vi "TREE_Get Sub Items.vi"(8 "error in":errorcluster, 10 "Par Tag":string, 11 "TreeRef":refnum<vi>) -> (0 "error out":errorcluster, 1 "Items":string[](array[string]), 2 "Tags":string[](array[string]), 3 "TreeRef":refnum<vi>)   [LabVIEW 2016]
doc: "Get sub items through input parent tag."
panel:
  # "Input"
  # "Output"
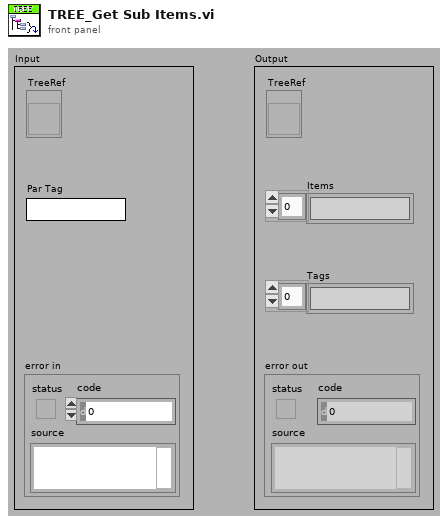
[diagram p1: front panel]
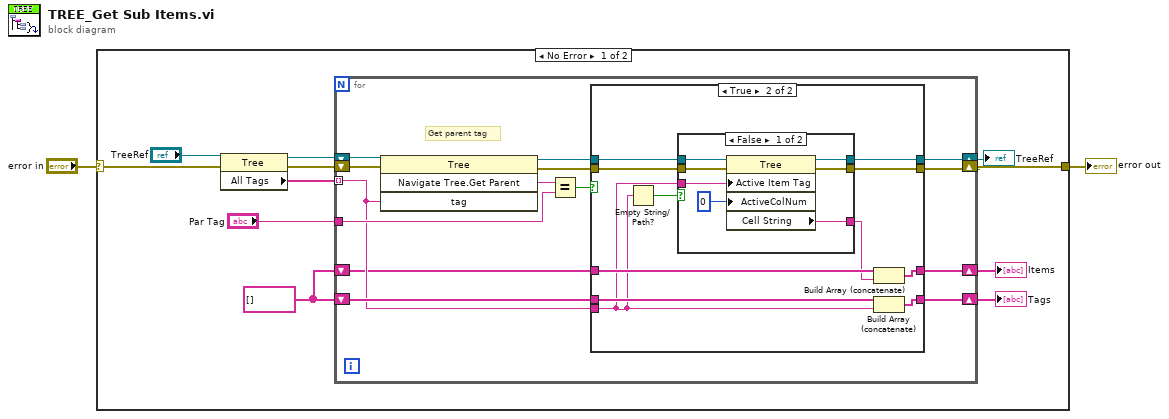
[diagram p0: block diagram]
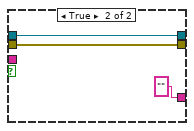
[diagram p3: hidden frame]
diagram:
  n1 = case shown="No Error" "error in" {
    selector: "error in" -> [w5 w53]
    tunnel: [w4 w53] -> w1
    frame No Error {
      w3 = string[] []
      n2 = property class="Tree"(reference="TreeRef", error in=w5) -> (reference out=w11:refnum<vi>, error out=w10:errorcluster, "All Tags"=w12:string[])
      n3 = for {
        tunnel: w12 -> [w21] mode=indexing
        tunnel: "Par Tag" -> [w24]
        shift-right: [w20] -> w6
        shift-left: w3 -> [w22]
        shift-right: [w16] -> w7
        shift-left: w3 -> [w17]
        shift-right: [w15] -> w8
        shift-left: w11 -> [w26]
        shift-right: [w14] -> w4
        shift-left: w10 -> [w27]
        # "Get parent tag"
        n4 = invoke class="Tree" method="Navigate Tree.Get Parent"(reference=w26, error in=w27, "tag"=w21) -> (reference out=w19:refnum<vi>, error out=w18:errorcluster, "Navigate Tree:Get Parent"=w25:string)  [unwired: 1 in, 1 out]
        n5 = Equal?(x=w25, y=w24) -> (x = y?=w23:bool)
        n6 = case shown="True" w23 {
          tunnel: w22 -> [w31 w42]
          tunnel: w21 -> [_ w38]
          tunnel: [w31 w41] -> w20
          tunnel: w19 -> [w29 w35]
          tunnel: w18 -> [w28 w36]
          tunnel: w17 -> [w30 w40]
          tunnel: [w30 w39] -> w16
          tunnel: [w29 w34] -> w15
          tunnel: [w28 w32] -> w14
          frame False {
          }
          frame True {
            n7 = Empty String/Path?(string/path=w38) -> (empty?=w37:bool)
            n8 = case shown="False" w37 {
              tunnel: [w49 w51] -> w32
              tunnel: [w48 w52] -> w34
              tunnel: w35 -> [w47 w52]
              tunnel: w36 -> [w46 w51]
              tunnel: [w45 "" ("Cell String")] -> w33
              tunnel: w38 -> [w43 _]
              frame False {
                n9 = property class="Tree"(reference=w47, error in=w46, "Active Item Tag"=w43, "ActiveColNum"=0 ("Active Cell:Active Column Number")) -> (reference out=w48:refnum<vi>, error out=w49:errorcluster, "Cell String"=w45:string)
              }
              frame True {
              }
            }
            n10 = Build Array (concatenate)(w40, w33) -> (w39:string[])
            n11 = Build Array (concatenate)(w42, w38) -> (w41:string[])
          }
        }
      }
      "TreeRef" <- w8
      "Items" <- w7
      "Tags" <- w6
    }
    frame Error {
    }
  }
  "error out" <- w1
